vi "FilterSet.vi"(8 "error in (no error)":errorcluster caption="错误输入（无错误）", 11 "ParamIn":cluster{"mode":u8, "AccCode":u32, "AccMask":u32}={"mode"=1, "AccCode"=0, "AccMask"=4294967295} {"AccMask" format="%08x"; "AccCode" format="%08x"; "mode" items=["接收所有类型"=1, "只接收标准帧"=2, "只接收扩展帧"=3]}) -> (0 "error out":errorcluster caption="错误输出", 2 "Cancel？":bool, 3 "ParamOut":cluster{"mode":u8, "AccCode":u32, "AccMask":u32}={"mode"=1, "AccCode"=0, "AccMask"=0} {"AccMask" format="%08x"; "AccCode" format="%08x"; "mode" items=["接收所有类型"=1, "只接收标准帧"=2, "只接收扩展帧"=3]})   [LabVIEW 2011]
panel:
  in  "calc":bool
  in  "cancel":bool
  in  "ok":bool
  in  "AccMask":u32 caption="屏蔽码：0x" format="%08x"
  in  "AccCode":u32 caption="验收码：0x" format="%08x"
  in  "mode":u8(ring)=1 caption="滤波方式：" items=["接收所有类型"=1, "只接收标准帧"=2, "只接收扩展帧"=3]
  in  "selfdef":bool
  out "tab":enum32{"标准ID", "扩展ID", "全ID"}(tab)
  in  "ID00":bool
  in  "ID01":bool
  in  "ID02":bool
  in  "ID03":bool
  in  "ID04":bool
  in  "ID05":bool
  in  "ID06":bool
  in  "ID07":bool
  in  "ID08":bool
  in  "ID09":bool
  in  "ID10":bool
  in  "t1":i32(listbox)=-1
  in  "EID17":bool
  in  "EID16":bool
  in  "EID15":bool
  in  "EID14":bool
  in  "EID13":bool
  in  "EID12":bool
  in  "EID11":bool
  in  "EID10":bool
  in  "EID09":bool
  in  "EID08":bool
  in  "EID07":bool
  in  "EID06":bool
  in  "EID05":bool
  in  "EID04":bool
  in  "EID03":bool
  in  "EID02":bool
  in  "EID01":bool
  in  "EID00":bool
  in  "EID26":bool
  in  "EID25":bool
  in  "EID24":bool
  in  "EID23":bool
  in  "EID22":bool
  in  "EID21":bool
  in  "EID20":bool
  in  "EID19":bool
  in  "EID18":bool
  in  "EID27":bool
  in  "EID28":bool
  in  "t2":i32(listbox)=-1
  in  "ID10 2":bool
  in  "ID09 2":bool
  in  "ID08 2":bool
  in  "ID07 2":bool
  in  "ID06 2":bool
  in  "ID05 2":bool
  in  "ID04 2":bool
  in  "ID03 2":bool
  in  "ID02 2":bool
  in  "ID01 2":bool
  in  "ID00 2":bool
  in  "EID17 2":bool
  in  "EID16 2":bool
  in  "EID15 2":bool
  in  "EID14 2":bool
  in  "EID13 2":bool
  in  "EID12 2":bool
  in  "EID11 2":bool
  in  "EID10 2":bool
  in  "EID09 2":bool
  in  "EID08 2":bool
  in  "EID07 2":bool
  in  "EID06 2":bool
  in  "EID05 2":bool
  in  "EID04 2":bool
  in  "EID03 2":bool
  in  "EID02 2":bool
  in  "EID01 2":bool
  in  "EID00 2":bool
  in  "EID26 2":bool
  in  "EID25 2":bool
  in  "EID24 2":bool
  in  "EID23 2":bool
  in  "EID22 2":bool
  in  "EID21 2":bool
  in  "EID20 2":bool
  in  "EID19 2":bool
  in  "EID18 2":bool
  in  "EID27 2":bool
  in  "EID28 2":bool
  in  "t3":i32(listbox)=-1
  in  "Submit":bool
  in  "IDSet":u32 caption="指定ID：0x" format="%x"
  in  "FilterMode":T1(ring) caption="滤波模式选择："
  # "注：如果对应位按钮显示为“X”表示此位为无关位，比如“XXX XXXXX111”，则表示收到的帧ID中只要低3位不为\n“111”就会被过滤掉。"
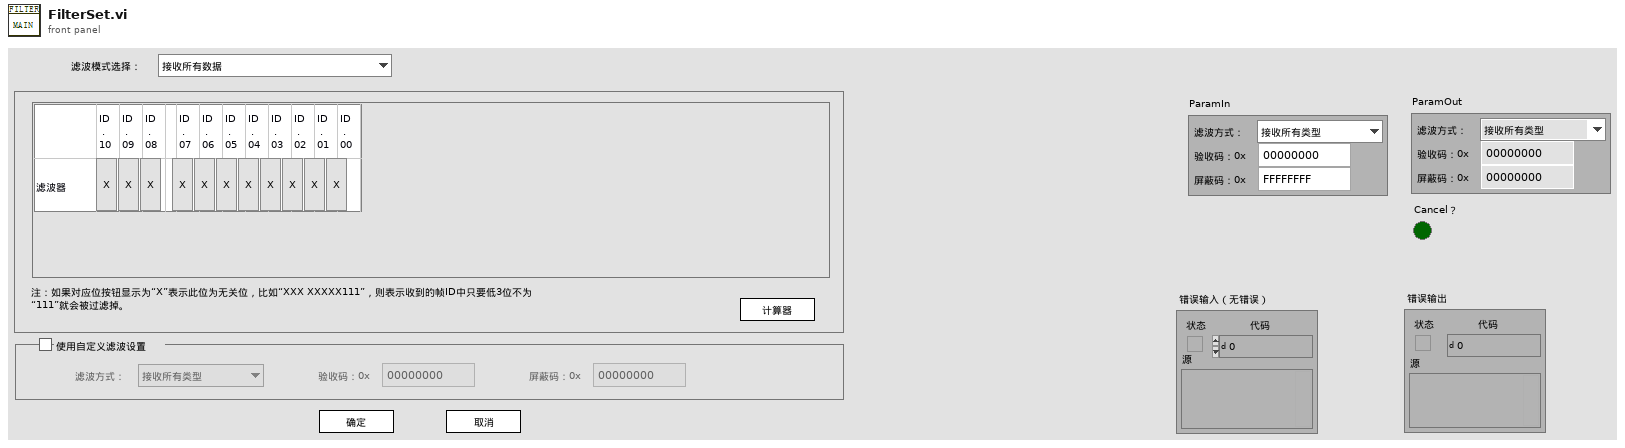
[diagram p1: front panel]
types:
  T1 = enum16{"接收所有数据", "标准帧滤波（设定接收单个ID）", "扩展帧滤波（设定接收单个ID）", "标准帧滤波（仅ID，自由设定）", "扩展帧滤波（仅ID，自由设定）"}
  T2 = cluster{"FilterMode":refnum<vi>, "IDSet":refnum<vi>, "t1":refnum<vi>, "t2":refnum<vi>, "t3":refnum<vi>, "Submit":refnum<vi>, "tab":refnum<vi>, "calc":refnum<vi>, "selfdef":refnum<vi>, "mode":refnum<vi>, "AccCode":refnum<vi>, "AccMask":refnum<vi>, "ok":refnum<vi>, "cancel":refnum<vi>}
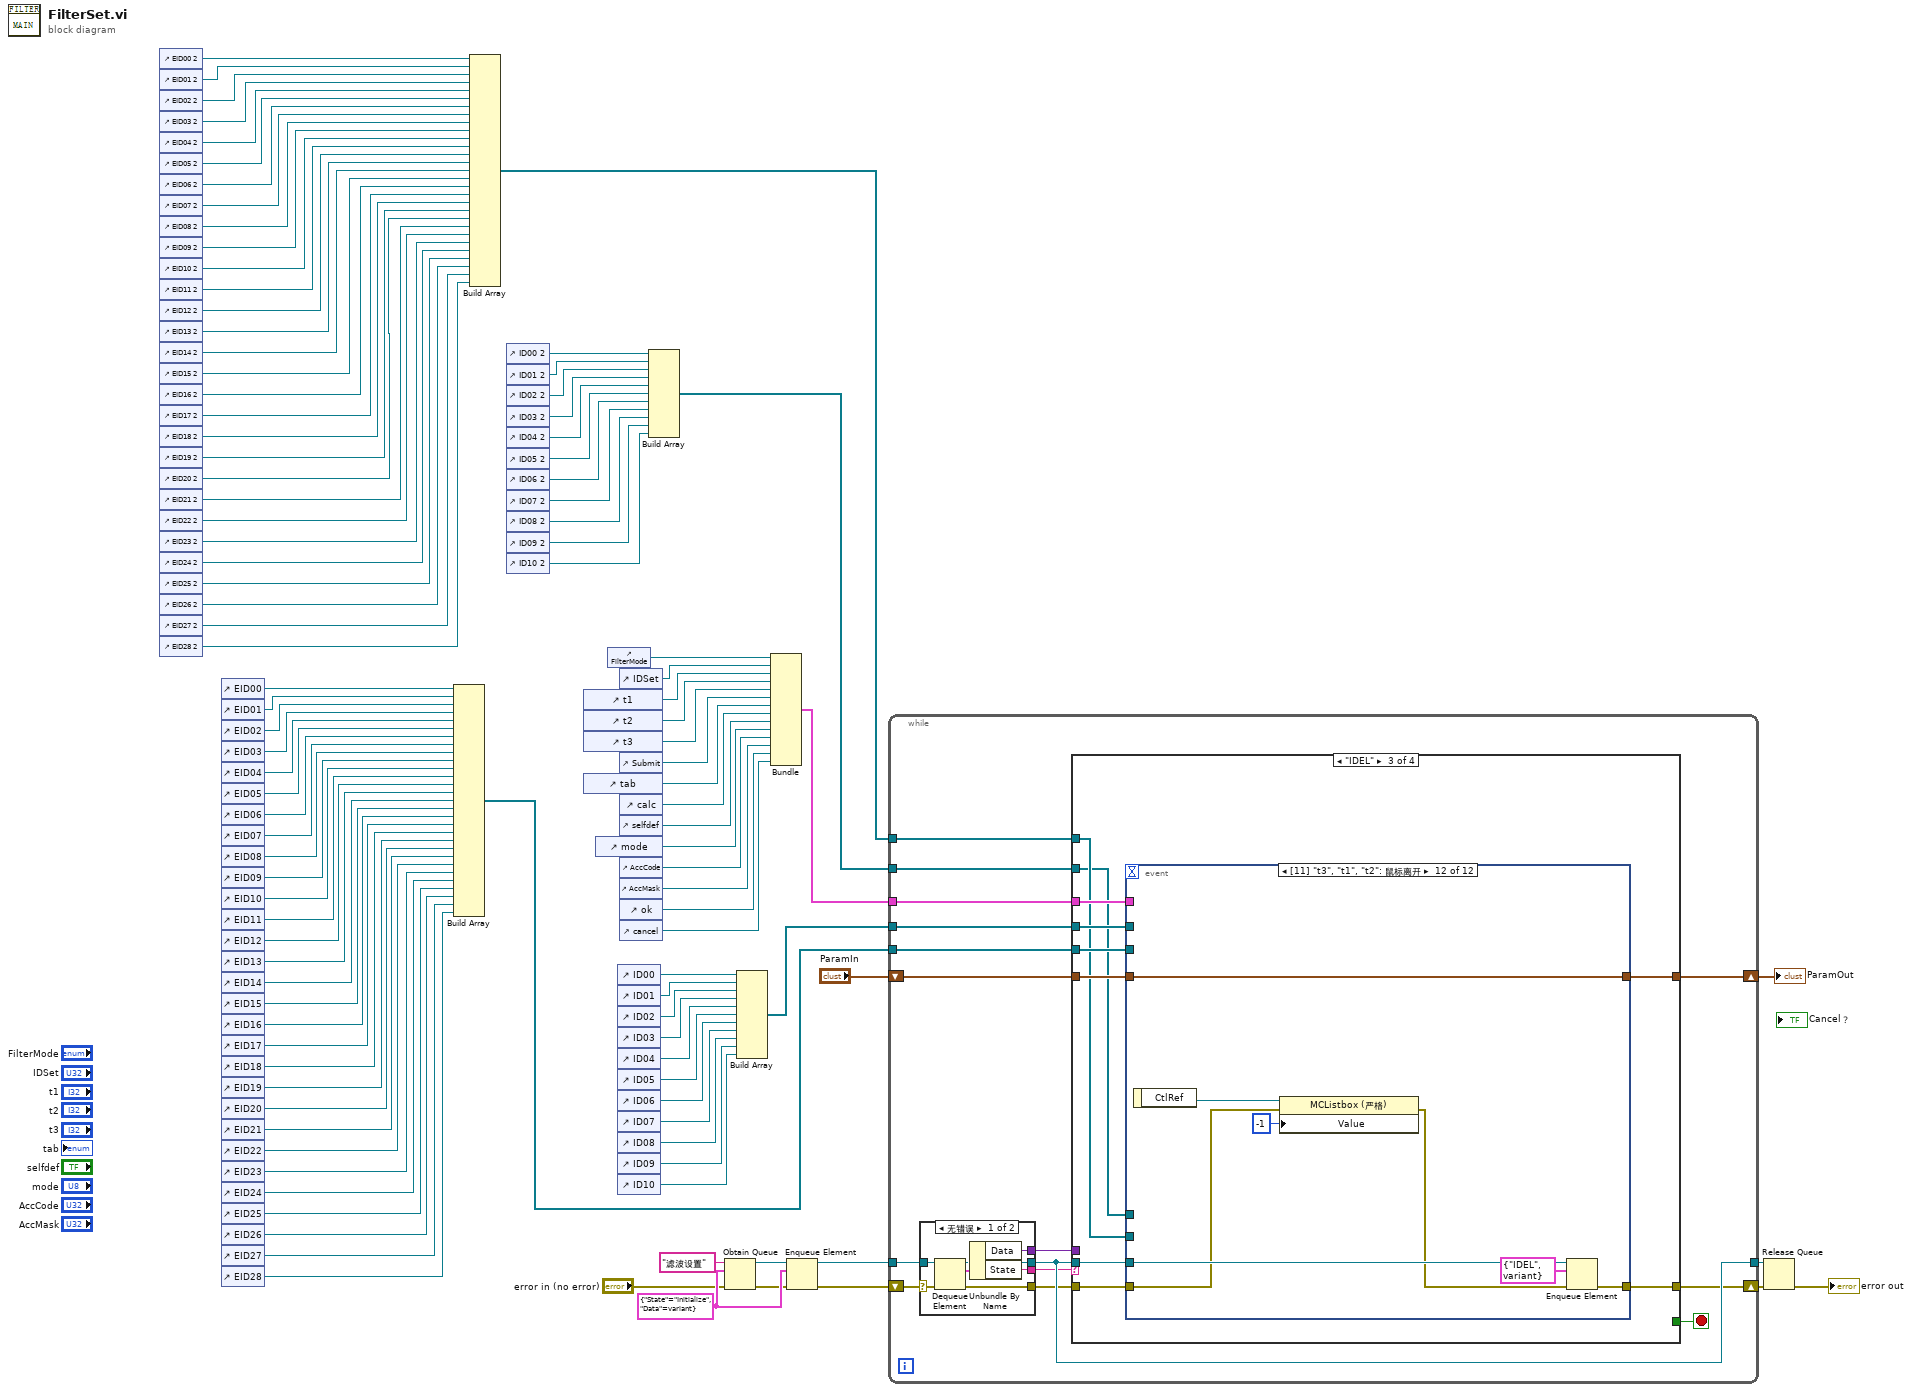
[diagram p0: block diagram]
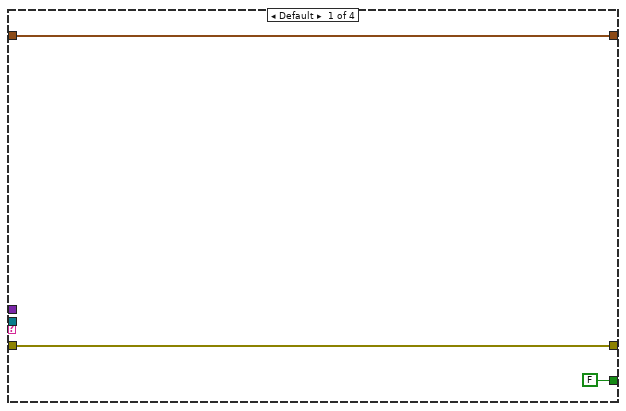
[diagram p2: hidden frame]
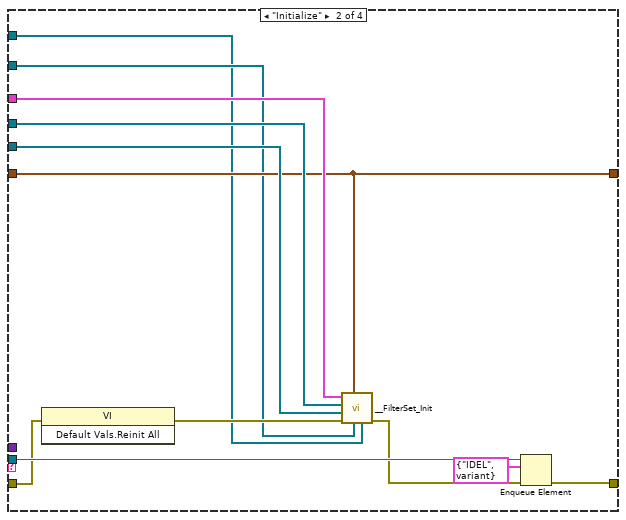
[diagram p3: hidden frame]
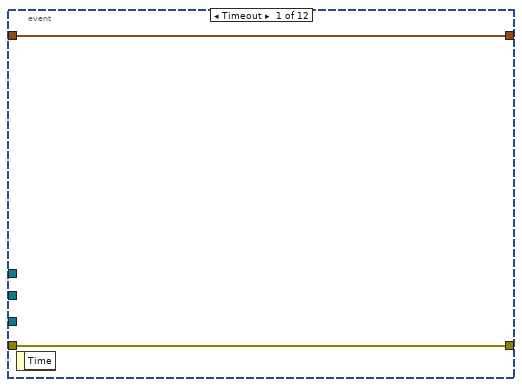
[diagram p4: hidden frame]
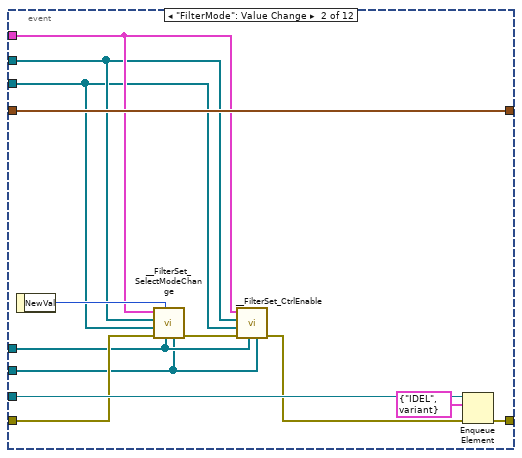
[diagram p5: hidden frame]
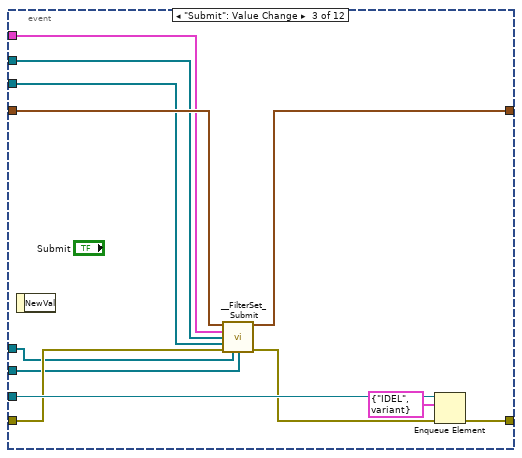
[diagram p6: hidden frame]
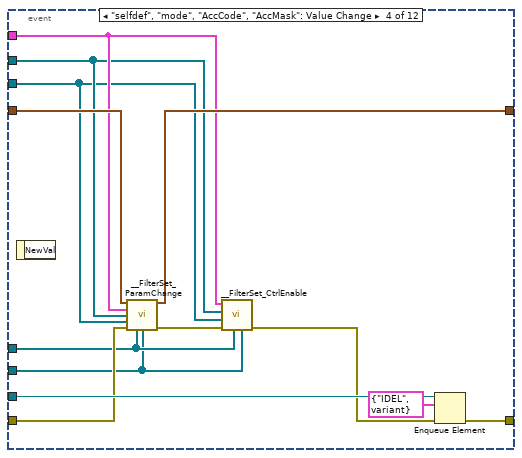
[diagram p7: hidden frame]
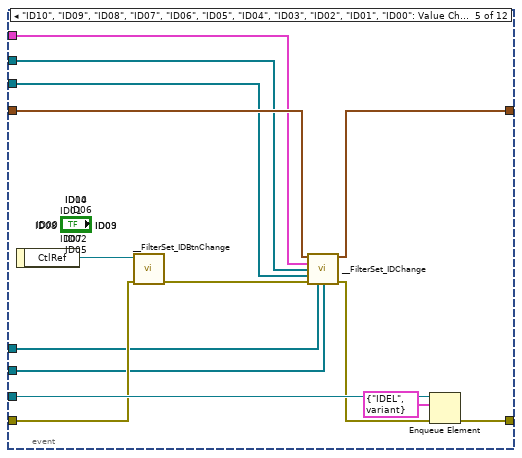
[diagram p8: hidden frame]
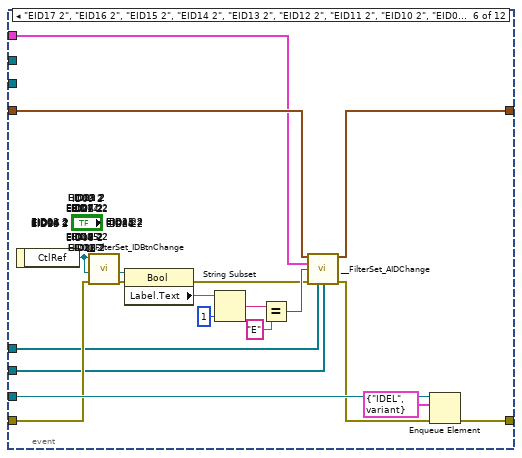
[diagram p9: hidden frame]
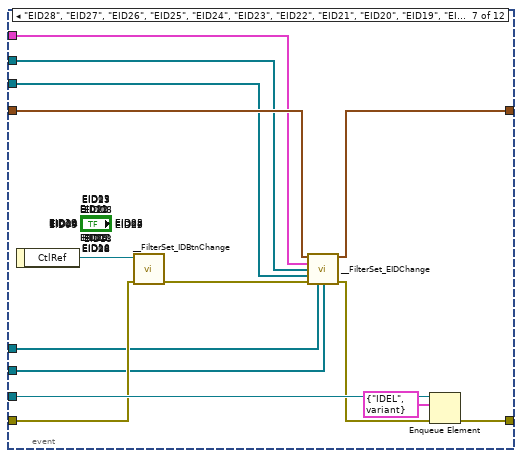
[diagram p10: hidden frame]
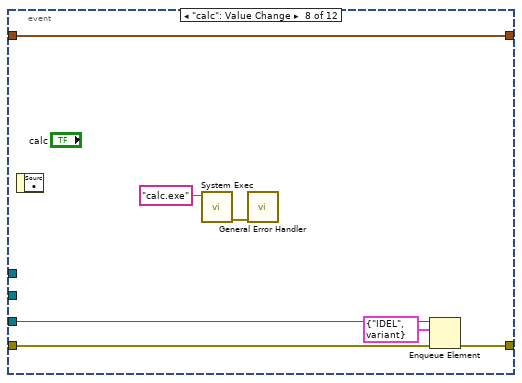
[diagram p11: hidden frame]
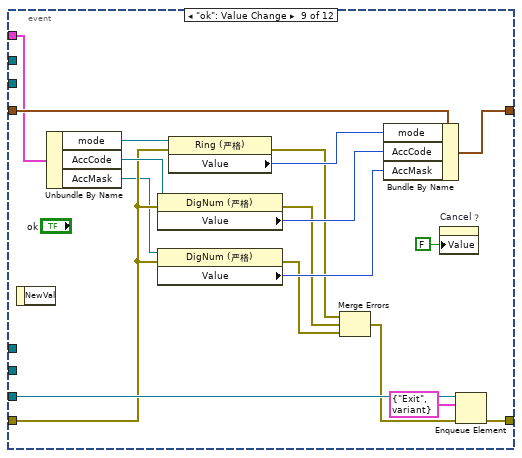
[diagram p12: hidden frame]
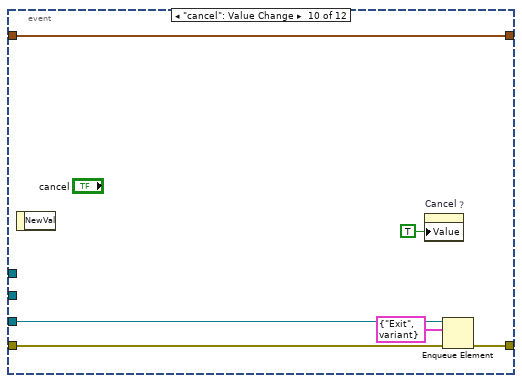
[diagram p13: hidden frame]
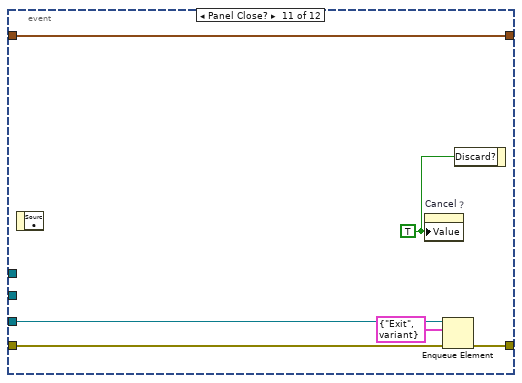
[diagram p14: hidden frame]
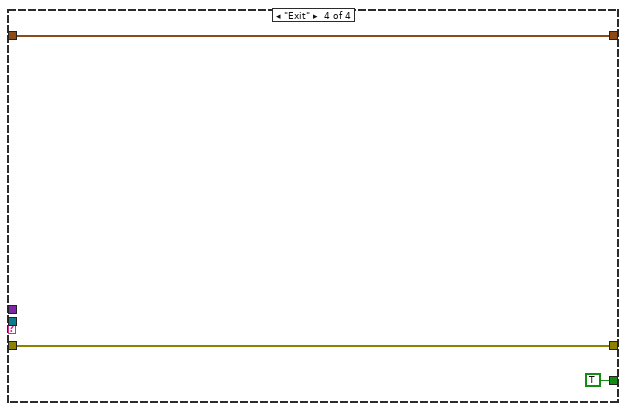
[diagram p15: hidden frame]
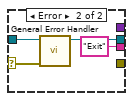
[diagram p16: hidden frame]
diagram:
  w111 = cluster{"State":string, "Data":variant} {"State"="Initialize", "Data"=variant}
  n1 = control-ref of="EID00 2"() -> (w45:refnum<vi>)
  n2 = control-ref of="EID01 2"() -> (w44:refnum<vi>)
  n3 = control-ref of="EID02 2"() -> (w43:refnum<vi>)
  n4 = control-ref of="EID03 2"() -> (w42:refnum<vi>)
  n5 = control-ref of="EID04 2"() -> (w41:refnum<vi>)
  n6 = control-ref of="EID05 2"() -> (w40:refnum<vi>)
  n7 = control-ref of="EID06 2"() -> (w39:refnum<vi>)
  n8 = control-ref of="EID07 2"() -> (w38:refnum<vi>)
  n9 = control-ref of="EID08 2"() -> (w37:refnum<vi>)
  n10 = control-ref of="EID09 2"() -> (w36:refnum<vi>)
  n11 = control-ref of="EID10 2"() -> (w35:refnum<vi>)
  n12 = control-ref of="EID11 2"() -> (w34:refnum<vi>)
  n13 = control-ref of="EID12 2"() -> (w33:refnum<vi>)
  n14 = control-ref of="EID13 2"() -> (w32:refnum<vi>)
  n15 = control-ref of="EID14 2"() -> (w31:refnum<vi>)
  n16 = control-ref of="EID15 2"() -> (w30:refnum<vi>)
  n17 = control-ref of="EID16 2"() -> (w29:refnum<vi>)
  n18 = control-ref of="EID17 2"() -> (w28:refnum<vi>)
  n19 = control-ref of="EID18 2"() -> (w27:refnum<vi>)
  n20 = control-ref of="EID19 2"() -> (w26:refnum<vi>)
  n21 = control-ref of="EID20 2"() -> (w25:refnum<vi>)
  n22 = control-ref of="EID21 2"() -> (w24:refnum<vi>)
  n23 = control-ref of="EID22 2"() -> (w23:refnum<vi>)
  n24 = control-ref of="EID23 2"() -> (w22:refnum<vi>)
  n25 = control-ref of="EID24 2"() -> (w21:refnum<vi>)
  n26 = control-ref of="EID25 2"() -> (w20:refnum<vi>)
  n27 = control-ref of="EID26 2"() -> (w19:refnum<vi>)
  n28 = control-ref of="EID27 2"() -> (w18:refnum<vi>)
  n29 = control-ref of="EID28 2"() -> (w17:refnum<vi>)
  n30 = control-ref of="EID00"() -> (w79:refnum<vi>)
  n31 = control-ref of="EID01"() -> (w78:refnum<vi>)
  n32 = control-ref of="EID02"() -> (w77:refnum<vi>)
  n33 = control-ref of="EID03"() -> (w76:refnum<vi>)
  n34 = control-ref of="EID04"() -> (w75:refnum<vi>)
  n35 = control-ref of="EID05"() -> (w74:refnum<vi>)
  n36 = control-ref of="EID06"() -> (w73:refnum<vi>)
  n37 = control-ref of="EID07"() -> (w72:refnum<vi>)
  n38 = control-ref of="EID08"() -> (w71:refnum<vi>)
  n39 = control-ref of="EID09"() -> (w70:refnum<vi>)
  n40 = control-ref of="EID10"() -> (w69:refnum<vi>)
  n41 = control-ref of="EID11"() -> (w68:refnum<vi>)
  n42 = control-ref of="EID12"() -> (w67:refnum<vi>)
  n43 = control-ref of="EID13"() -> (w66:refnum<vi>)
  n44 = control-ref of="EID14"() -> (w65:refnum<vi>)
  n45 = control-ref of="EID15"() -> (w64:refnum<vi>)
  n46 = control-ref of="EID16"() -> (w63:refnum<vi>)
  n47 = control-ref of="EID17"() -> (w62:refnum<vi>)
  n48 = control-ref of="EID18"() -> (w61:refnum<vi>)
  n49 = control-ref of="EID19"() -> (w60:refnum<vi>)
  n50 = control-ref of="EID20"() -> (w59:refnum<vi>)
  n51 = control-ref of="EID21"() -> (w58:refnum<vi>)
  n52 = control-ref of="EID22"() -> (w57:refnum<vi>)
  n53 = control-ref of="EID23"() -> (w56:refnum<vi>)
  n54 = control-ref of="EID24"() -> (w55:refnum<vi>)
  n55 = control-ref of="EID25"() -> (w54:refnum<vi>)
  n56 = control-ref of="EID26"() -> (w53:refnum<vi>)
  n57 = control-ref of="EID27"() -> (w52:refnum<vi>)
  n58 = control-ref of="EID28"() -> (w51:refnum<vi>)
  n59 = Build Array(w79, w78, w77, w76, w75, w74, w73, w72, w71, w70, w69, w68, w67, w66, w65, w64, w63, w62, w61, w60, w59, w58, w57, w56, w55, w54, w53, w52, w51) -> (w48:refnum<vi>[])
  n60 = Build Array(w45, w44, w43, w42, w41, w40, w39, w38, w37, w36, w35, w34, w33, w32, w31, w30, w29, w28, w27, w26, w25, w24, w23, w22, w21, w20, w19, w18, w17) -> (w5:refnum<vi>[])
  n61 = control-ref of="ID00 2"() -> (w16:refnum<vi>)
  n62 = control-ref of="ID01 2"() -> (w15:refnum<vi>)
  n63 = control-ref of="ID02 2"() -> (w14:refnum<vi>)
  n64 = control-ref of="ID03 2"() -> (w13:refnum<vi>)
  n65 = control-ref of="ID04 2"() -> (w12:refnum<vi>)
  n66 = control-ref of="ID05 2"() -> (w11:refnum<vi>)
  n67 = control-ref of="ID06 2"() -> (w10:refnum<vi>)
  n68 = control-ref of="ID07 2"() -> (w9:refnum<vi>)
  n69 = control-ref of="ID08 2"() -> (w8:refnum<vi>)
  n70 = control-ref of="ID09 2"() -> (w7:refnum<vi>)
  n71 = control-ref of="ID10 2"() -> (w6:refnum<vi>)
  n72 = control-ref of="t1"() -> (w101:refnum<vi>)
  n73 = control-ref of="t2"() -> (w100:refnum<vi>)
  n74 = control-ref of="t3"() -> (w3:refnum<vi>)
  n75 = control-ref of="tab"() -> (w98:refnum<vi>)
  n76 = control-ref of="mode"() -> (w95:refnum<vi>)
  n77 = control-ref of="FilterMode"() -> (w103:refnum<vi>)
  n78 = control-ref of="ID00"() -> (w90:refnum<vi>)
  n79 = control-ref of="ID01"() -> (w89:refnum<vi>)
  n80 = control-ref of="ID02"() -> (w88:refnum<vi>)
  n81 = control-ref of="ID03"() -> (w87:refnum<vi>)
  n82 = control-ref of="ID04"() -> (w86:refnum<vi>)
  n83 = control-ref of="ID05"() -> (w85:refnum<vi>)
  n84 = control-ref of="ID06"() -> (w84:refnum<vi>)
  n85 = control-ref of="ID07"() -> (w83:refnum<vi>)
  n86 = control-ref of="ID08"() -> (w82:refnum<vi>)
  n87 = control-ref of="ID09"() -> (w81:refnum<vi>)
  n88 = control-ref of="ID10"() -> (w80:refnum<vi>)
  n89 = control-ref of="IDSet"() -> (w102:refnum<vi>)
  n90 = control-ref of="Submit"() -> (w99:refnum<vi>)
  n91 = control-ref of="calc"() -> (w97:refnum<vi>)
  n92 = control-ref of="selfdef"() -> (w96:refnum<vi>)
  n93 = control-ref of="AccCode"() -> (w94:refnum<vi>)
  n94 = control-ref of="AccMask"() -> (w93:refnum<vi>)
  n95 = control-ref of="ok"() -> (w92:refnum<vi>)
  n96 = control-ref of="cancel"() -> (w91:refnum<vi>)
  n97 = Build Array(w16, w15, w14, w13, w12, w11, w10, w9, w8, w7, w6) -> (w4:refnum<vi>[])
  n98 = Obtain Queue(name (unnamed)="滤波设置", element data type=w111, error in (no error)="error in (no error)") -> (queue out=w109:refnum<queue>, error out=w110:errorcluster)  [unwired: 2 in, 1 out]
  n99 = Build Array(w90, w89, w88, w87, w86, w85, w84, w83, w82, w81, w80) -> (w49:refnum<vi>[])
  n100 = Bundle("FilterMode"=w103, "IDSet"=w102, "t1"=w101, "t2"=w100, "t3"=w3, "Submit"=w99, "tab"=w98, "calc"=w97, "selfdef"=w96, "mode"=w95, "AccCode"=w94, "AccMask"=w93, "ok"=w92, "cancel"=w91) -> (w50:T2)  [unwired: 1 in]
  n101 = Enqueue Element(queue=w109, element=w111, error in (no error)=w110) -> (queue out=w106:refnum<queue>, error out=w107:errorcluster)  [unwired: 2 out]
  n102 = while {
    shift-right: [w121] -> w105
    shift-left: w107 -> [w125]
    tunnel: w106 -> [w124]
    tunnel: [w126] -> w104
    tunnel: w50 -> [w119]
    tunnel: w49 -> [w118]
    tunnel: w48 -> [w117]
    shift-right: [w116] -> w47
    shift-left: "ParamIn" -> [w115]
    tunnel: w5 -> [w113]
    tunnel: w4 -> [w112]
    stop <- w120 stop-if-true
    n103 = case shown="无错误" w125 {
      selector: w125 -> [w291 w295]
      tunnel: w124 -> [w292 w294]
      tunnel: [w287 "Exit" ("State")] -> w123
      tunnel: [w289 _] -> w122
      tunnel: [w288 w294] -> w126
      tunnel: [w286 _] -> w114
      frame No Error {
        n104 = Dequeue Element(queue=w292, error in (no error)=w291) -> (queue out=w288:refnum<queue>, element=w290:cluster{"State":string, "Data":variant}, error out=w289:errorcluster)  [unwired: 2 out]
        n105 = Unbundle By Name(w290) -> ("Data"=w286:variant, "State"=w287:string)
      }
      frame Error {
        n106 = call <vilib>:"General Error Handler.vi"("error in (no error)"=w295) -> ()  [unwired: 1 in, 14 out]
      }
    }
    n107 = case shown="\"IDEL\"" w123 {
      tunnel: w122 -> [w129 w138 w151 w285]
      tunnel: [w129 w139 w150 w285] -> w121
      tunnel: [FALSE _ _ TRUE] -> w120
      tunnel: w126 -> [_ w140 w149 _]
      tunnel: w119 -> [_ w136 w148 _]
      tunnel: w118 -> [_ w135 w147 _]
      tunnel: w117 -> [_ w134 w146 _]
      tunnel: [w127 w133 w144 w283] -> w116
      tunnel: w115 -> [w127 w133 w145 w283]
      tunnel: w114 -> [_ _ _ _]
      tunnel: w113 -> [_ w130 w143 _]
      tunnel: w112 -> [_ w131 w142 _]
      frame Default {
      }
      frame "Initialize" {
        n108 = invoke class="VI" method="Default Vals.Reinit All"(error in=w138) -> (error out=w137:errorcluster)  [unwired: 2 in, 2 out]
        n109 = call "__FilterSet_Init.vi"("EIDRef 2"=w130, "IDRef 2"=w131, "ParamIn"=w133, "error in (no error)"=w137, "EIDRef"=w134, "IDRef"=w135, "CtrlRef"=w136) -> ("error out"=w132:errorcluster)  [unwired: 4 in]
        n110 = Enqueue Element(queue=w140, element=cluster{"State":string, "Data":variant} {"State"="IDEL", "Data"=variant}, error in (no error)=w132) -> (error out=w139:errorcluster)  [unwired: 3 out]
      }
      frame "IDEL" {
        n111 = event shown="[11] \"t3\", \"t1\", \"t2\": 鼠标离开" {
          selector: _ -> [_ _ _ _ _ _ _ _ _ _ _ _]
          dyn-events: _ -> [_ _ _ _ _ _ _ _ _ _ _ _]
          timeout: _ -> [_ _ _ _ _ _ _ _ _ _ _ _]
          tunnel: w151 -> [w153 w163 w175 w186 w195 w216 w227 w239 w251 w265 w271 w277]
          tunnel: [w153 w165 w177 w190 w204 w222 w236 w243 w261 w266 w272 w280] -> w150
          tunnel: w149 -> [_ w166 w176 w189 w203 w221 w235 w242 w260 w264 w270 w279]
          tunnel: w148 -> [_ w158 w171 w183 w199 w217 w231 _ w256 _ _ _]
          tunnel: w147 -> [_ w157 w170 w182 w198 _ w230 _ _ _ _ _]
          tunnel: w146 -> [_ w156 w169 w181 w197 _ w229 _ _ _ _ _]
          tunnel: w145 -> [w152 w161 w173 w185 w202 w220 w234 w241 w258 w268 w274 w282]
          tunnel: [w152 w161 w172 w184 w201 w219 w233 w241 w257 w268 w274 w282] -> w144
          tunnel: w143 -> [_ w154 w167 w179 w192 w214 w224 _ _ _ _ _]
          tunnel: w142 -> [_ w155 w168 w180 w193 w215 w225 _ _ _ _ _]
          event Timeout {
            n112 = event-data() -> ()  [unwired: 1 in, 1 out]
          }
          event "FilterMode": Value Change {
            n113 = event-data() -> ("NewVal"=w162:T1)  [unwired: 1 in]
            n114 = call "__FilterSet_SelectModeChange.vi"("EIDRef 2"=w154, "IDRef 2"=w155, "Mode"=w162, "error in (no error)"=w163, "EIDRef"=w156, "IDRef"=w157, "CtrlRef"=w158) -> ("error out"=w160:errorcluster)  [unwired: 4 in]
            n115 = call "__FilterSet_CtrlEnable.vi"("EIDRef 2"=w154, "IDRef 2"=w155, "error in (no error)"=w160, "EIDRef"=w156, "IDRef"=w157, "CtrlRef"=w158) -> ("error out"=w159:errorcluster)  [unwired: 5 in]
            n116 = Enqueue Element(queue=w166, element=cluster{"State":string, "Data":variant} {"State"="IDEL", "Data"=variant}, error in (no error)=w159) -> (error out=w165:errorcluster)  [unwired: 3 out]
          }
          event "Submit": Value Change {
            n117 = event-data() -> ()  [unwired: 1 in, 1 out]
            n118 = call "__FilterSet_Submit.vi"("Param in"=w173, "CtrlRef"=w171, "IDRef"=w170, "EIDRef"=w169, "error in (no error)"=w175, "IDRef 2"=w168, "EIDRef 2"=w167) -> ("Param out"=w172:cluster{"mode":u8, "AccCode":u32, "AccMask":u32}, "error out"=w174:errorcluster)  [unwired: 7 in]
            n119 = Enqueue Element(queue=w176, element=cluster{"State":string, "Data":variant} {"State"="IDEL", "Data"=variant}, error in (no error)=w174) -> (error out=w177:errorcluster)  [unwired: 3 out]
          }
          event "selfdef", "mode", "AccCode", "AccMask": Value Change {
            n120 = event-data() -> ()  [unwired: 1 in, 1 out]
            n121 = call "__FilterSet_ParamChange.vi"("Param in"=w185, "CtrlRef"=w183, "IDRef"=w182, "EIDRef"=w181, "error in (no error)"=w186, "IDRef 2"=w180, "EIDRef 2"=w179) -> ("Param out"=w184:cluster{"mode":u8, "AccCode":u32, "AccMask":u32}, "error out"=w187:errorcluster)  [unwired: 7 in]
            n122 = call "__FilterSet_CtrlEnable.vi"("EIDRef 2"=w179, "IDRef 2"=w180, "error in (no error)"=w187, "EIDRef"=w181, "IDRef"=w182, "CtrlRef"=w183) -> ("error out"=w188:errorcluster)  [unwired: 5 in]
            n123 = Enqueue Element(queue=w189, element=cluster{"State":string, "Data":variant} {"State"="IDEL", "Data"=variant}, error in (no error)=w188) -> (error out=w190:errorcluster)  [unwired: 3 out]
          }
          event "ID10", "ID09", "ID08", "ID07", "ID06", "ID05", "ID04", "ID03", "ID02", "ID01", "ID00": Value Change {
            n124 = event-data() -> ("CtlRef"=w196:refnum<vi>)  [unwired: 1 in]
            n125 = call "__FilterSet_IDBtnChange.vi"("error in (no error)"=w195, "Btn Ref"=w196) -> ("error out"=w194:errorcluster)  [unwired: 9 in]
            n126 = call "__FilterSet_IDChange.vi"("Param in"=w202, "CtrlRef"=w199, "IDRef"=w198, "EIDRef"=w197, "error in (no error)"=w194, "IDRef 2"=w193, "EIDRef 2"=w192) -> ("Param out"=w201:cluster{"mode":u8, "AccCode":u32, "AccMask":u32}, "error out"=w200:errorcluster)  [unwired: 7 in]
            n127 = Enqueue Element(queue=w203, element=cluster{"State":string, "Data":variant} {"State"="IDEL", "Data"=variant}, error in (no error)=w200) -> (error out=w204:errorcluster)  [unwired: 3 out]
          }
          event "EID17 2", "EID16 2", "EID15 2", "EID14 2", "EID13 2", "EID12 2", "EID11 2", "EID10 2", "EID09 2", "EID08 2", "EID07 2", "EID06 2", "EID05 2", "EID04 2", "EID03 2", "EID02 2", "EID01 2", "EID00 2", "EID26 2", "EID25 2", "EID24 2", "EID23 2", "EID22 2", "EID21 2", "EID20 2", "EID19 2", "EID18 2", "EID27 2", "EID28 2", "ID10 2", "ID09 2", "ID08 2", "ID07 2", "ID06 2", "ID05 2", "ID04 2", "ID03 2", "ID02 2", "ID01 2", "ID00 2": Value Change {
            n128 = event-data() -> ("CtlRef"=w206:refnum<vi>)  [unwired: 1 in]
            n129 = call "__FilterSet_IDBtnChange.vi"("error in (no error)"=w216, "Btn Ref"=w206) -> ("error out"=w213:errorcluster)  [unwired: 9 in]
            n130 = property class="Bool"(reference=w206, error in=w213) -> (error out=w207:errorcluster, "Label.Text"=w212:string)  [unwired: 1 out]
            n131 = String Subset(string=w212, length (rest)=1 ("长度（剩余）")) -> (substring=w210:string)  [unwired: 1 in]
            n132 = Equal?(x=w210, y="E") -> (x = y?=w208:bool)
            n133 = call "__FilterSet_AIDChange.vi"("Param in"=w220, "CtrlRef"=w217, "EID?"=w208, "error in (no error)"=w207, "IDRef 2"=w215, "EIDRef 2"=w214) -> ("Param out"=w219:cluster{"mode":u8, "AccCode":u32, "AccMask":u32}, "error out"=w218:errorcluster)  [unwired: 8 in]
            n134 = Enqueue Element(queue=w221, element=cluster{"State":string, "Data":variant} {"State"="IDEL", "Data"=variant}, error in (no error)=w218) -> (error out=w222:errorcluster)  [unwired: 3 out]
          }
          event "EID28", "EID27", "EID26", "EID25", "EID24", "EID23", "EID22", "EID21", "EID20", "EID19", "EID18", "EID17", "EID16", "EID15", "EID14", "EID13", "EID12", "EID11", "EID10", "EID09", "EID08", "EID07", "EID06", "EID05", "EID04", "EID03", "EID02", "EID01", "EID00": Value Change {
            n135 = event-data() -> ("CtlRef"=w228:refnum<vi>)  [unwired: 1 in]
            n136 = call "__FilterSet_IDBtnChange.vi"("error in (no error)"=w227, "Btn Ref"=w228) -> ("error out"=w226:errorcluster)  [unwired: 9 in]
            n137 = call "__FilterSet_EIDChange.vi"("Param in"=w234, "CtrlRef"=w231, "IDRef"=w230, "EIDRef"=w229, "error in (no error)"=w226, "IDRef 2"=w225, "EIDRef 2"=w224) -> ("Param out"=w233:cluster{"mode":u8, "AccCode":u32, "AccMask":u32}, "error out"=w232:errorcluster)  [unwired: 7 in]
            n138 = Enqueue Element(queue=w235, element=cluster{"State":string, "Data":variant} {"State"="IDEL", "Data"=variant}, error in (no error)=w232) -> (error out=w236:errorcluster)  [unwired: 3 out]
          }
          event "calc": Value Change {
            n139 = event-data() -> ()  [unwired: 1 in, 1 out]
            n140 = call <vilib>:"System Exec.vi"("command line"="calc.exe") -> ("error out"=w238:errorcluster)  [unwired: 7 in, 3 out]
            n141 = call <vilib>:"General Error Handler.vi"("error in (no error)"=w238) -> ()  [unwired: 1 in, 14 out]
            n142 = Enqueue Element(queue=w242, element=cluster{"State":string, "Data":variant} {"State"="IDEL", "Data"=variant}, error in (no error)=w239) -> (error out=w243:errorcluster)  [unwired: 3 out]
          }
          event "ok": Value Change {
            n143 = event-data() -> ()  [unwired: 1 in, 1 out]
            n144 = Unbundle By Name(w256) -> ("mode"=w255:refnum<vi>, "AccCode"=w253:refnum<vi>, "AccMask"=w250:refnum<vi>)
            n145 = property class="DigNum (严格)"(reference=w253, error in=w251) -> (error out=w247:errorcluster, "Value"=w252:u32)  [unwired: 1 out]
            n146 = property class="DigNum (严格)"(reference=w250, error in=w251) -> (error out=w246:errorcluster, "Value"=w249:u32)  [unwired: 1 out]
            n147 = property class="Ring (严格)"(reference=w255, error in=w251) -> (error out=w248:errorcluster, "Value"=w254:u8)  [unwired: 1 out]
            n148 = Merge Errors(w248, w247, w246) -> (w245:errorcluster)
            n149 = Bundle By Name(cluster=w258, "mode"=w254, "AccCode"=w252, "AccMask"=w249) -> (w257:cluster{"mode":u8, "AccCode":u32, "AccMask":u32})
            n150 = property on="Cancel？" class="Bool (严格)"("Value"=FALSE ("Cancel？")) -> ()  [unwired: 2 in, 2 out]
            n151 = Enqueue Element(queue=w260, element=cluster{"State":string, "Data":variant} {"State"="Exit", "Data"=variant}, error in (no error)=w245) -> (error out=w261:errorcluster)  [unwired: 3 out]
          }
          event "cancel": Value Change {
            n152 = event-data() -> ()  [unwired: 1 in, 1 out]
            n153 = property on="Cancel？" class="Bool (严格)"("Value"=TRUE ("Cancel？")) -> ()  [unwired: 2 in, 2 out]
            n154 = Enqueue Element(queue=w264, element=cluster{"State":string, "Data":variant} {"State"="Exit", "Data"=variant}, error in (no error)=w265) -> (error out=w266:errorcluster)  [unwired: 3 out]
          }
          event Panel Close? {
            w269 = TRUE ("Cancel？")
            n155 = event-data() -> ()  [unwired: 1 in, 1 out]
            n156 = property on="Cancel？" class="Bool (严格)"("Value"=w269) -> ()  [unwired: 2 in, 2 out]
            n157 = Enqueue Element(queue=w270, element=cluster{"State":string, "Data":variant} {"State"="Exit", "Data"=variant}, error in (no error)=w271) -> (error out=w272:errorcluster)  [unwired: 3 out]
            n158 = event-data("Discard?"=w269) -> ()  [unwired: 1 in, 1 out]
          }
          event "t3", "t1", "t2": Mouse Leave {
            n159 = event-data() -> ("CtlRef"=w278:refnum<vi>)  [unwired: 1 in]
            n160 = property class="MCListbox (严格)"(reference=w278, error in=w277, "Value"=-1 ("值")) -> (error out=w276:errorcluster)  [unwired: 1 out]
            n161 = Enqueue Element(queue=w279, element=cluster{"State":string, "Data":variant} {"State"="IDEL", "Data"=variant}, error in (no error)=w276) -> (error out=w280:errorcluster)  [unwired: 3 out]
          }
        }
      }
      frame "Exit" {
      }
    }
  }
  "ParamOut" <- w47
  n162 = Release Queue(queue=w104, error in (no error)=w105) -> (error out=→"error out":errorcluster)  [unwired: 3 out]
